vi "Increment Bearing.vi"(8 "Error In":errorcluster, 10 "Increment Value":dbl, 11 "Bearing":dbl) -> (0 "Error Out":errorcluster, 3 "New Bearing":dbl)   [LabVIEW 2014]
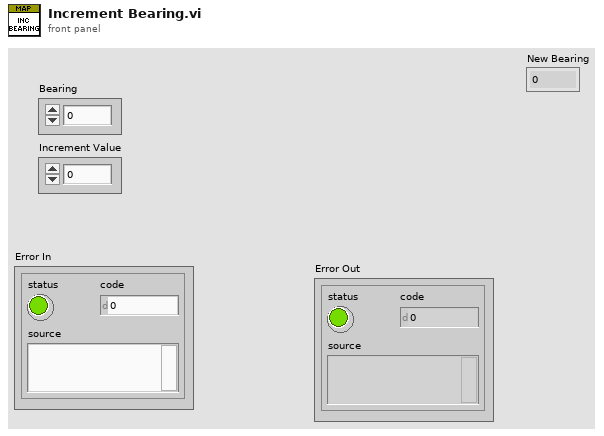
[diagram p1: front panel]
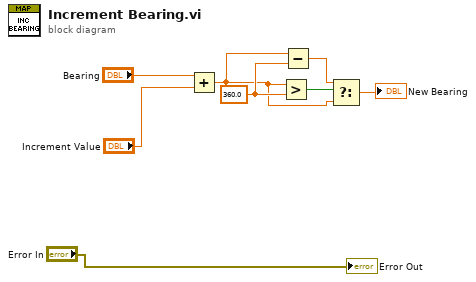
[diagram p0: block diagram]
diagram:
  w5 = 360.0 ("y")
  n1 = Add(x="Bearing", y="Increment Value") -> (x+y=w3:dbl)
  n2 = Greater?(x=w3, y=w5) -> (0:w6:bool)
  n3 = Subtract(x=w3, y=w5) -> (x-y=w4:dbl)
  n4 = Select(t=w4, s=w6, f=w3) -> (s? t:f=→"New Bearing":dbl)
  "Error Out" <- "Error In"
